vi "get available methods.vi"(8 "error in":errorcluster, 9 "invoke_node_id":string) -> (0 "error out":errorcluster, 3 "All Supported Methods":T1)   [LabVIEW 2020]
doc: "Returns the available methods for an Invoke Node as a list of {Unique ID string, Data name, Short name (localized), Long name (localized)} objects. \n\nUse this before set_invoke_node to find the correct method — pass the \"Unique ID string\" value (not \"Data name\") as set_invoke_node's method_name for a reliable exact match. \n\nMake sure a concrete-class reference (VI, Control, Application, etc.) is already wired into the Invoke Node's input, since the available methods depend on that class."
uses:
  <vilib>/_script/All Supported PropertiesOrMethods TypeDefs/ASPM_ArrayOfUniqueIDStringDatanameShortnameLongname.ctl
  <vilib>/_script/All Supported PropertiesOrMethods TypeDefs/ASPM_UniqueIDStringDatanameShortnameLongname.ctl
  G-AI Core/G-AI Core.lvlib
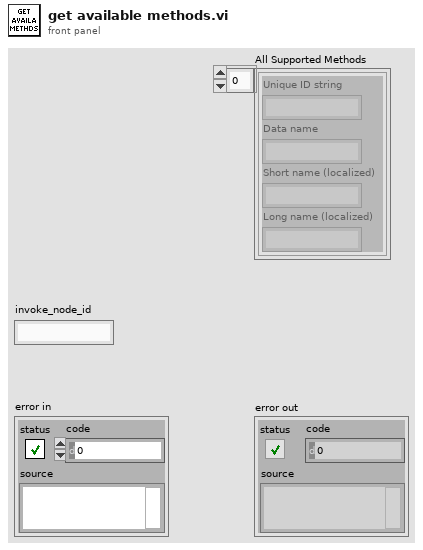
[diagram p1: front panel]
types:
  T1 = typedef "ASPM_ArrayOfUniqueIDStringDatanameShortnameLongname.ctl" = T2[]
  T2 = typedef "ASPM_UniqueIDStringDatanameShortnameLongname.ctl" = cluster{"Unique ID string":string, "Data name":string, "Short name (localized)":string, "Long name (localized)":string}
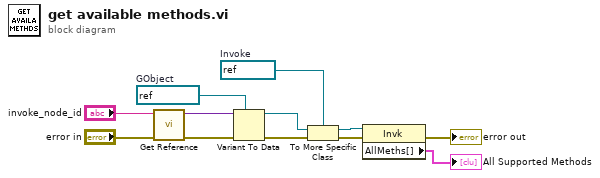
[diagram p0: block diagram]
diagram:
  w7 = refnum<vi> refnum  # Invoke
  w8 = refnum<vi> refnum  # GObject
  n1 = call "Get Reference.vi"("error in"="error in", "id"="invoke_node_id") -> ("error out"=w11:errorcluster, "reference"=w10:variant)  [unwired: 8 in]
  n2 = Variant To Data(error in=w11, type=w8, Variant=w10) -> (data=w6:refnum<vi>, error out=w9:errorcluster)
  n3 = To More Specific Class(target class=w7, reference=w6, error in=w9) -> (specific class reference=w3:refnum<vi>, error out=w5:errorcluster)
  n4 = property class="Invk"(reference=w3, error in=w5) -> (error out=→"error out":errorcluster, "AllMeths[]"=→"All Supported Methods":T1)  [unwired: 1 out]
